vi "Write Value.vi"(8 "error in (no error)":errorcluster, 9 "Value":string, 10 "Name":string, 11 "Session in":refnum<class "Session.lvclass">) -> (0 "error out":errorcluster, 2 "Value Replaced?":bool, 3 "Session out":refnum<class "Session.lvclass">)   [LabVIEW 2020, in "HTTP Server.lvlib" / "Session.lvclass"]
uses:
  Session.lvclass
  Session.lvclass/Session.ctl
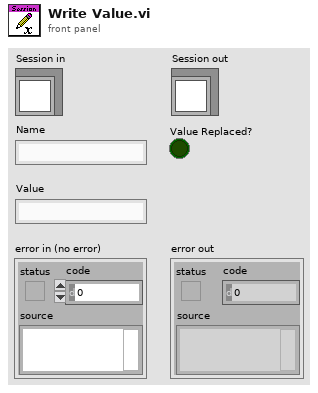
[diagram p1: front panel]
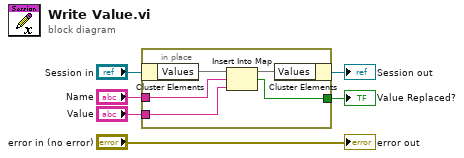
[diagram p0: block diagram]
diagram:
  n1 = in-place {
    in-place-border: "Name" -> [w10]
    in-place-border: "Value" -> [w9]
    in-place-border: [w7] -> w1
    n2 = in-place-cluster #1("Session in") -> ("Values"=w11:map{string, string})
    n3 = Insert Into Map(map in=w11, key=w10, value=w9) -> (map out=w8:map{string, string}, key already included?=w7:bool)  [unwired: 1 out]
    n4 = in-place-cluster #1("Values"=w8) -> (→"Session out":refnum<class "Session.lvclass">)
  }
  "Value Replaced?" <- w1
  "error out" <- "error in (no error)"
